vi "写入Allowed VI Alias.vi"(8 "error in (no error)":errorcluster caption="错误输入（无错误）", 9 "Allowed VI Path":path[](array[path]), 10 "Allowed VI Alias":string[](array[string]), 11 "PanelDataNode输入":refnum<class "PanelDataNode.lvclass">) -> (0 "error out":errorcluster caption="错误输出", 3 "PanelDataNode输出":refnum<class "PanelDataNode.lvclass">)   [LabVIEW 2016, in "PanelDataNode.lvclass"]
uses:
  PanelDataNode.lvclass
  PanelDataNode.lvclass/PanelDataNode.ctl
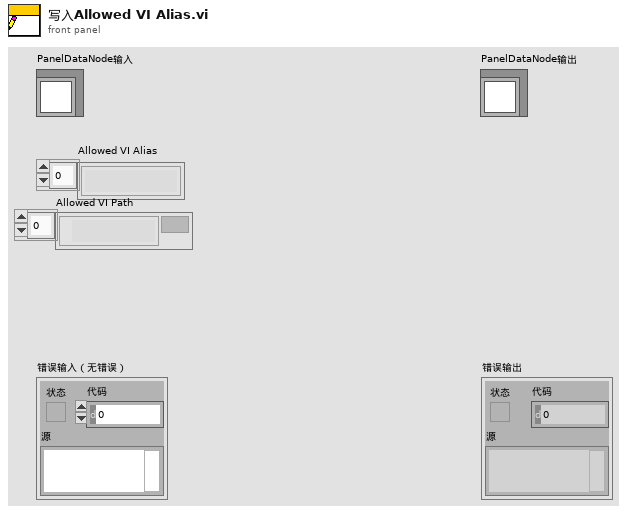
[diagram p1: front panel]
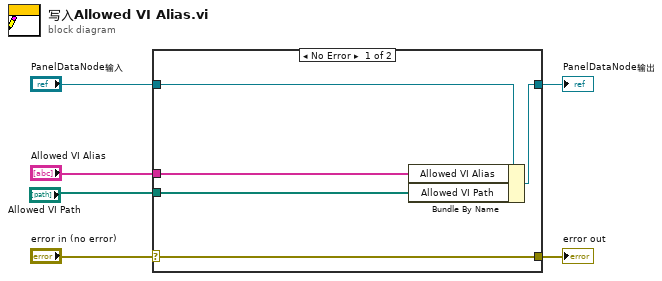
[diagram p0: block diagram]
diagram:
  n1 = case shown="No Error" "error in (no error)" {
    selector: "error in (no error)" -> [w11 w12]
    tunnel: [w11 w12] -> w5
    tunnel: [w9 w13] -> w3
    tunnel: "PanelDataNode输入" -> [w10 w13]
    tunnel: "Allowed VI Alias" -> [w8 _]
    tunnel: "Allowed VI Path" -> [w7 _]
    frame No Error {
      n2 = Bundle By Name(cluster=w10, "Allowed VI Alias"=w8, "Allowed VI Path"=w7) -> (w9:refnum<class "PanelDataNode.lvclass">)
    }
    frame Error {
    }
  }
  "error out" <- w5
  "PanelDataNode输出" <- w3
